vi "CameraViewerDaft.vi"() -> ()   [LabVIEW 2017]
uses:
  <vilib>/userdefined/High Color/IMAQdx.ctl
  <vilib>/vision/driver/IMAQdx.llb/IMAQdx Camera Control Mode.ctl
  <vilib>/vision/driver/NI_Vision_Acquisition_Software.lvlib
panel:
  in  "Image Type":T1 items=["Grayscale (U8)", "Grayscale (I16)", "Grayscale (SGL)", "Complex (CSG)", "RGB (U32)", "HSL (U32)", "RGB (U64)", "Grayscale (U16)"]
  in  "Image Name":string="untitled"
  out "error out":errorcluster
  out "Image Out":T2(plugin-control)
  in  "stop":bool
  in  "Camera Control Mode":T3
  in  "Session In":T4
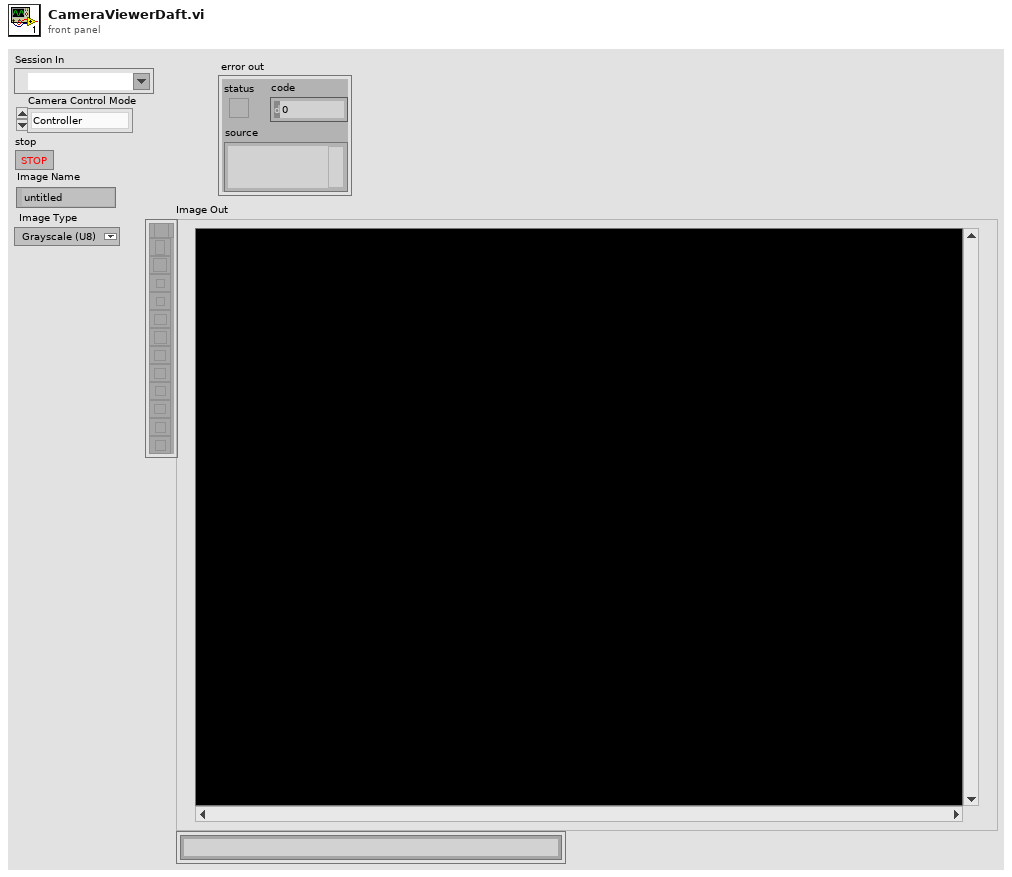
[diagram p1: front panel]
types:
  T1 = typedef "Image Type" = u32
  T2 = typedef "IMAQ Image.ctl" = refnum<image>
  T3 = typedef "NI_Vision_Acquisition_Software.lvlib/IMAQdx Camera Control Mode.ctl" = enum32{"Controller", "Listener"}
  T4 = typedef "IMAQdx.ctl" = refnum<k21>
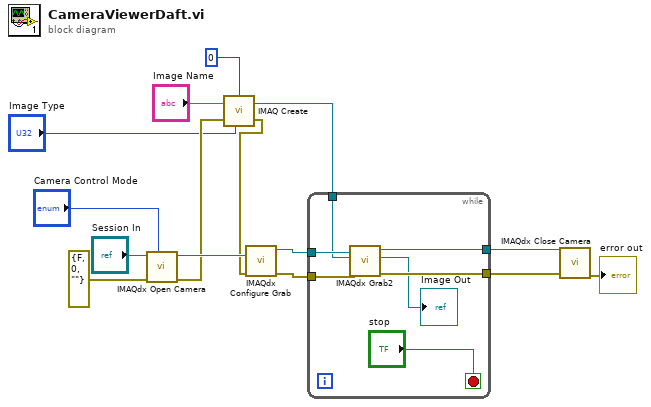
[diagram p0: block diagram]
diagram:
  n1 = call <vilib>:"IMAQdx Open Camera.vi"("Camera Control Mode"="Camera Control Mode", "error in"=errorcluster {"status"=FALSE, "code"=0, "source"=""}, "Session In"="Session In") -> ("error out"=w5:errorcluster, "Session Out"=w13:T4)  [unwired: 7 in]
  n2 = call "IMAQ Create"("Border Size"=0, "Image Name"="Image Name", "Image Type"="Image Type", "error in (no error)"=w5) -> ("New Image"=w3:T2, "error out"=w4:errorcluster)  [unwired: 1 in]
  n3 = call <vilib>:"IMAQdx Configure Grab.vi"("error in"=w4, "Session In"=w13) -> ("error out"=w11:errorcluster, "Session Out"=w12:T4)  [unwired: 8 in]
  n4 = while {
    tunnel: w12 -> [w22]
    tunnel: w11 -> [w21]
    tunnel: [w19] -> w10
    tunnel: [w18] -> w9
    tunnel: w3 -> [w16]
    stop <- "stop" stop-if-true
    n5 = call <vilib>:"IMAQdx Grab2.vi"("error in"=w21, "Image In"=w16, "Session In"=w22) -> ("error out"=w18:errorcluster, "Image Out"=→"Image Out":T2, "Session Out"=w19:T4)  [unwired: 5 in, 1 out]
  }
  n6 = call <vilib>:"IMAQdx Close Camera.vi"("error in"=w9, "Session In"=w10) -> ("error out"=→"error out":errorcluster)  [unwired: 9 in]
